vi "Configure Resistor Band Visibility.vi"(8 "error in (no error)":errorcluster, 10 "Number of Bands in":u8=4 min=3 max=6 step=1, 11 "Color Box Refnum":refnum<vi>[](array[refnum])) -> (0 "error out":errorcluster, 2 "Number of Bands out":u8=4 min=3 max=6 step=1)   [LabVIEW 2018, in "Front Panel Interface.lvlib"]
doc: "Configures the visibility of the resistor band ColorBox controls on the Front Panel according to the selected number of bands.\n\nThe VI receives the <b>Number of Bands</b> and an array of <b>ColorBox Refnums</b>. It determines which resistor bands must be visible for 3-, 4-, 5-, and 6-band resistor configurations and updates the <b>Visible</b> property of each ColorBox control.\n\nThe VI only configures Front Panel visibility. It does not modify the color or value of any resistor band."
uses:
  Front Panel Interface.lvlib
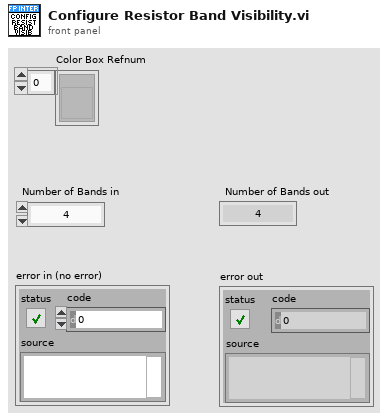
[diagram p1: front panel]
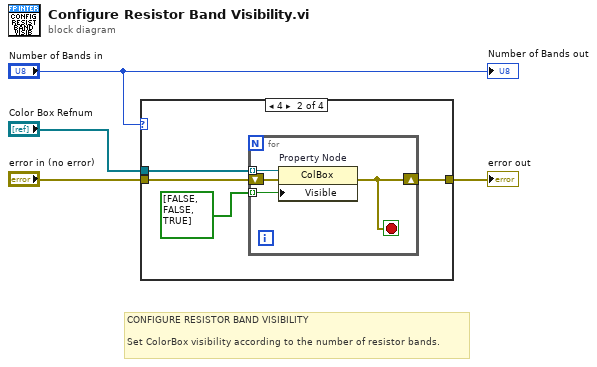
[diagram p0: block diagram]
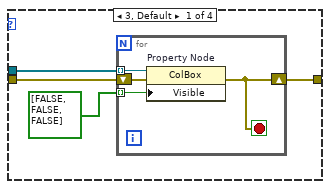
[diagram p2: hidden frame]
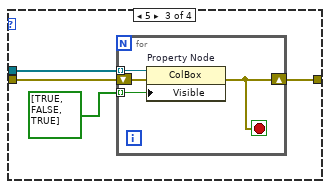
[diagram p3: hidden frame]
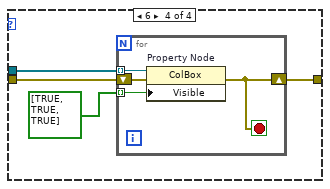
[diagram p4: hidden frame]
diagram:
  # "CONFIGURE RESISTOR BAND VISIBILITY\n\nSet ColorBox visibility according to the number of resistor bands."
  n1 = case shown="4" "Number of Bands in" {
    tunnel: "Color Box Refnum" -> [w8 w13 w24 w32]
    tunnel: [w6 w14 w21 w29] -> w4
    tunnel: "error in (no error)" -> [w5 w15 w22 w30]
    frame 3, Default {
      n2 = for {
        tunnel: w8 -> [w12] mode=indexing
        tunnel: bool[] [FALSE, FALSE, FALSE] -> [w11] mode=indexing
        shift-right: [w9] -> w6
        shift-left: w5 -> [w10]
        stop <- w9 stop-if-true
        n3 = property on="Property Node" class="ColBox"(reference=w12, error in=w10, "Visible"=w11) -> (error out=w9:errorcluster)  [unwired: 1 out]
      }
    }
    frame 4 {
      n4 = for {
        tunnel: w13 -> [w20] mode=indexing
        tunnel: bool[] [FALSE, FALSE, TRUE] -> [w19] mode=indexing
        shift-right: [w17] -> w14
        shift-left: w15 -> [w18]
        stop <- w17 stop-if-true
        n5 = property on="Property Node" class="ColBox"(reference=w20, error in=w18, "Visible"=w19) -> (error out=w17:errorcluster)  [unwired: 1 out]
      }
    }
    frame 5 {
      n6 = for {
        tunnel: w24 -> [w28] mode=indexing
        tunnel: bool[] [TRUE, FALSE, TRUE] -> [w27] mode=indexing
        shift-right: [w25] -> w21
        shift-left: w22 -> [w26]
        stop <- w25 stop-if-true
        n7 = property on="Property Node" class="ColBox"(reference=w28, error in=w26, "Visible"=w27) -> (error out=w25:errorcluster)  [unwired: 1 out]
      }
    }
    frame 6 {
      n8 = for {
        tunnel: w32 -> [w36] mode=indexing
        tunnel: bool[] [TRUE, TRUE, TRUE] -> [w35] mode=indexing
        shift-right: [w33] -> w29
        shift-left: w30 -> [w34]
        stop <- w33 stop-if-true
        n9 = property on="Property Node" class="ColBox"(reference=w36, error in=w34, "Visible"=w35) -> (error out=w33:errorcluster)  [unwired: 1 out]
      }
    }
  }
  "error out" <- w4
  "Number of Bands out" <- "Number of Bands in"
